vi "ST Status.vi"(5 "error in (no error)":errorcluster, 6 "VISA resource name":refnum<visa-resource-name>) -> (0 "error out":errorcluster, 1 "String Received":string, 2 "Result Code":i32, 3 "VISA resource name out":refnum<visa-resource-name>, 4 "Ready and OK":bool)   [LabVIEW 2009]
doc: "This VI will report the status of the Robot. The result out has the following meaning:\n 0 >>> Operation not complete\n 1 >>> Operation Complete with an Error\n 2 >>> Operation Complete without Error\n-1 >>> Operation caused a Communication Error"
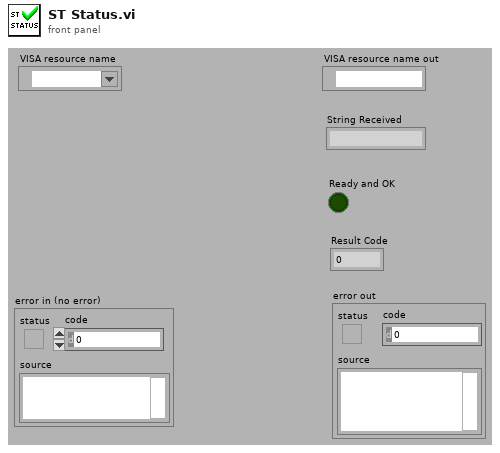
[diagram p1: front panel]
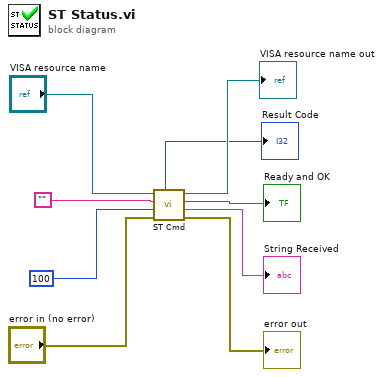
[diagram p0: block diagram]
diagram:
  n1 = call "ST Cmd.vi"("error in (no error)"="error in (no error)", "Time Out"=100, "Command String"="", "VISA resource name"="VISA resource name") -> ("error out"=→"error out":errorcluster, "String Received"=→"String Received":string, "Ready and OK"=→"Ready and OK":bool, "VISA resource name out"=→"VISA resource name out":refnum<visa-resource-name>, "Result Code"=→"Result Code":i32)
